vi "SetGXMLCfgFreq.vi"(8 "error in (no error)":errorcluster, 10 "FreqChanCfg":T1, 11 "Freq in":refnum<class "Frequency.lvclass">) -> (0 "error out":errorcluster, 3 "Freq out":refnum<class "Frequency.lvclass">)   [LabVIEW 2012, in "Measurement Channels.lvlib" / "Frequency.lvclass"]
uses:
  Frequency.lvclass
  FreqProps_TD.ctl
  Frequency.lvclass/Frequency.ctl
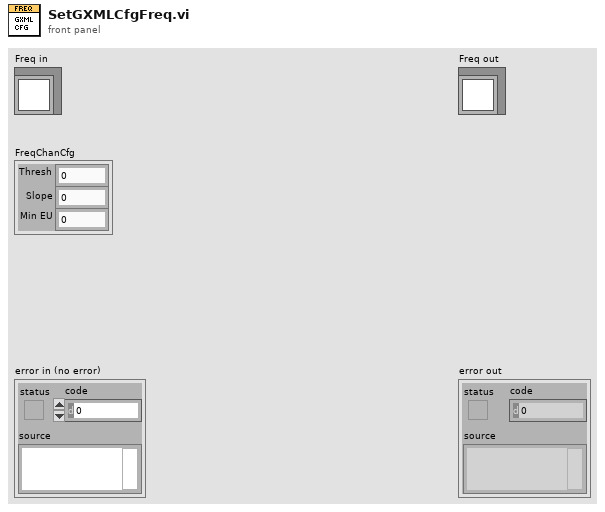
[diagram p1: front panel]
types:
  T1 = typedef "Measurement Channels.lvlib/Frequency.lvclass/FreqProps_TD.ctl" = cluster{"Thresh":dbl, "Slope":u16, "Min EU":dbl}
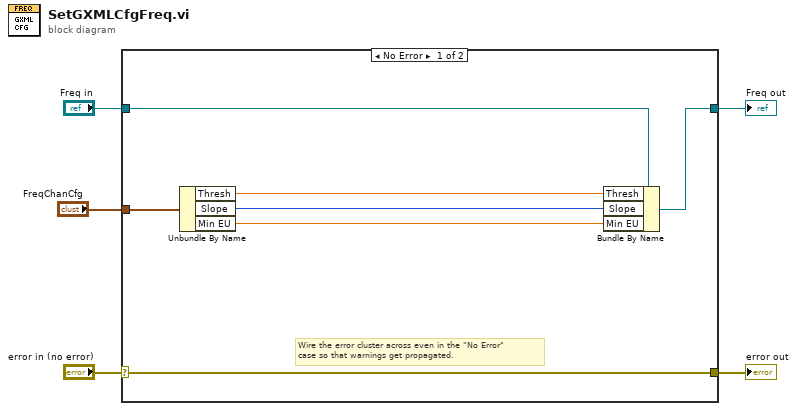
[diagram p0: block diagram]
diagram:
  n1 = case shown="No Error" "error in (no error)" {
    selector: "error in (no error)" -> [w12 w14]
    tunnel: [w12 w14] -> w4
    tunnel: [w6 w13] -> w2
    tunnel: "Freq in" -> [w7 w13]
    tunnel: "FreqChanCfg" -> [w8 _]
    frame No Error {
      # "Wire the error cluster across even in the \"No Error\"\ncase so that warnings get propagated."
      n2 = Unbundle By Name(w8) -> ("Thresh"=w11:dbl, "Slope"=w10:u16, "Min EU"=w9:dbl)
      n3 = Bundle By Name(cluster=w7, "Thresh"=w11, "Slope"=w10, "Min EU"=w9) -> (w6:refnum<class "Frequency.lvclass">)
    }
    frame Error {
    }
  }
  "error out" <- w4
  "Freq out" <- w2
